vi "EjercicioCase.vi"() -> ()   [LabVIEW 2022 SP3]
panel:
  in  "stop":bool
  in  "Enum (Operation)":T1(ring)
  out "Resultado":dbl
  in  "B":dbl
  in  "A":dbl
  # "Estructura Case"
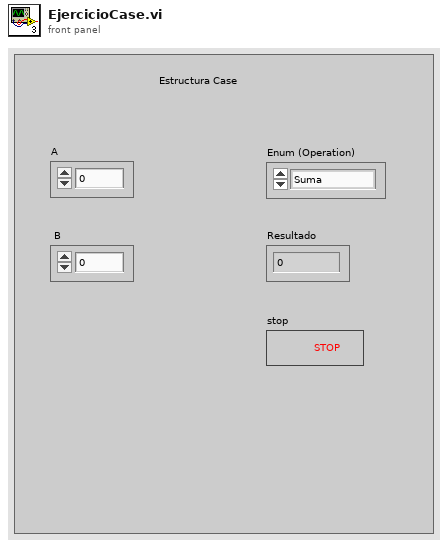
[diagram p1: front panel]
types:
  T1 = enum16{"Suma", "Resta", "Multiplicación", "División"}
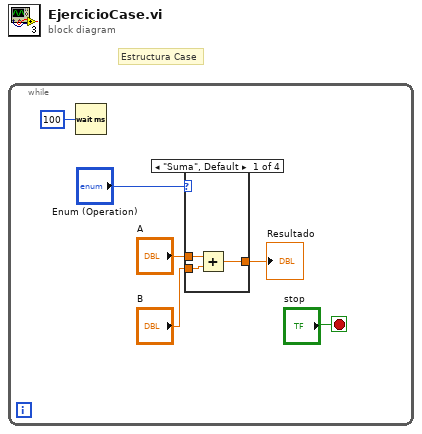
[diagram p0: block diagram]
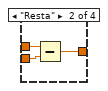
[diagram p2: hidden frame]
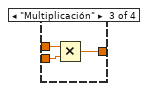
[diagram p3: hidden frame]
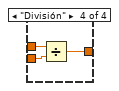
[diagram p4: hidden frame]
diagram:
  # "Estructura Case"
  n1 = while {
    stop <- "stop" stop-if-true
    n2 = Wait (ms)(milliseconds to wait=u32 100) -> ()  [unwired: 1 out]
    n3 = case shown="\"Suma\", Default" "Enum (Operation)" {
      tunnel: "A" -> [w9 w12 w15 w18]
      tunnel: "B" -> [w8 w11 w14 w17]
      tunnel: [w7 w10 w13 w16] -> w1
      frame "Suma", Default {
        n4 = Add(x=w9, y=w8) -> (x+y=w7:dbl)
      }
      frame "Resta" {
        n5 = Subtract(x=w12, y=w11) -> (x-y=w10:dbl)
      }
      frame "Multiplicación" {
        n6 = Multiply(x=w15, y=w14) -> (x*y=w13:dbl)
      }
      frame "División" {
        n7 = Divide(x=w18, y=w17) -> (x/y=w16:dbl)
      }
    }
    "Resultado" <- w1
  }
